vi "str_to_u32_arr.vi"(1 "string":string) -> (0 "array":u32[](array[numeric]))   [LabVIEW 2011]
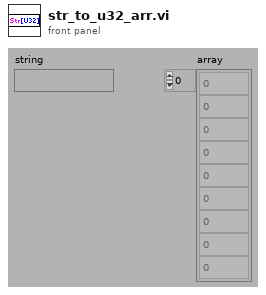
[diagram p1: front panel]
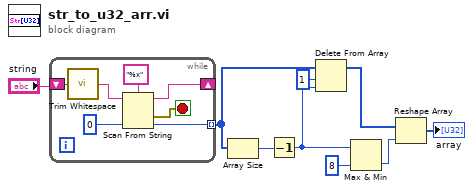
[diagram p0: block diagram]
diagram:
  n1 = while {
    shift-right: [w13] -> _
    shift-left: "string" -> [w16]
    tunnel: [w11] -> w5 mode=indexing
    stop <- w10 stop-if-true
    n2 = call <vilib>:"Trim Whitespace.vi"("string"=w16) -> ("trimmed string"=w15:string)  [unwired: 1 in]
    n3 = Scan From String(format string="%x" ("格式字符串"), input string=w15, default 1=u32 0) -> (remaining string=w13:string, error out=w10:errorcluster, output 1=w11:u32)  [unwired: 2 in, 1 out]
  }
  n4 = Array Size(array=w5) -> (size(s)=w3:i32)
  n5 = Decrement(x=w3) -> (x-1=w1:i32)
  n6 = Delete From Array(array=w5, length=1 ("长度"), index=w1) -> (array with subset deleted=w4:u32[])  [unwired: 1 out]
  n7 = Max & Min(x=w1, y=8 ("维数大小")) -> (min(x,y)=w6:i32)  [unwired: 1 out]
  n8 = Reshape Array(w4, w6) -> (→"array":u32[])
